vi "thermocouple-calibrate-average.vi"(11 "adam-chassis-all-data-out in":T1) -> (3 "adam-chassis-all-data-out out":T1)   [LabVIEW 2024]
uses:
  adam5000_LLB/controls/adam-5000-all-chassis-data.ctl
  adam5000_LLB/controls/adam-5000-all-module-datas.ctl
  adam5000_LLB/controls/digital-output-cluster.ctl
  adam5000_LLB/controls/digitial-input-cluster.ctl
  adam5000_LLB/controls/analog-output-cluster.ctl
  adam5000_LLB/controls/analog-input-cluster.ctl
  adam5000_LLB/controls/thermocouple-input-cluster.ctl
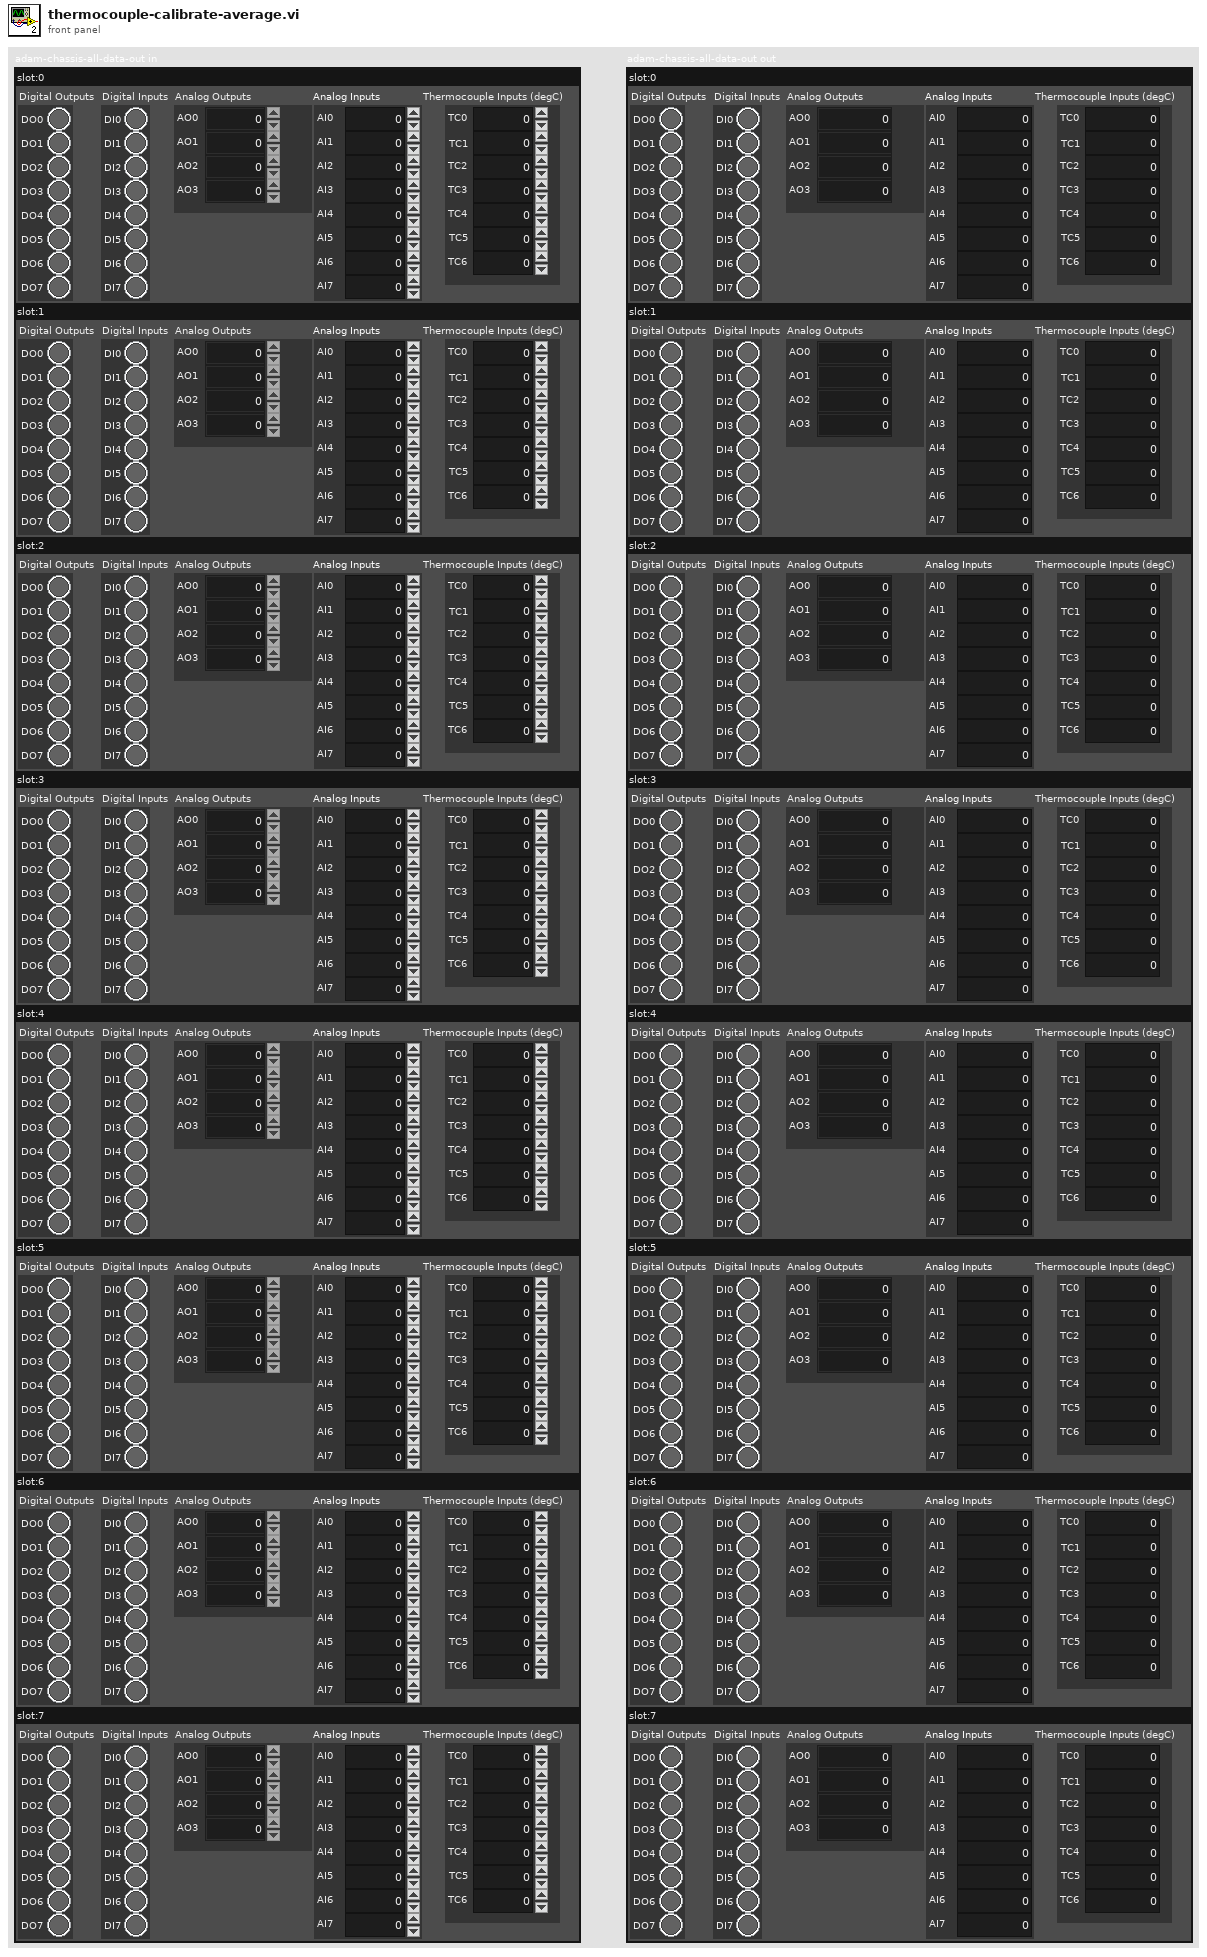
[diagram p1: front panel]
types:
  T1 = typedef "adam-5000-all-chassis-data.ctl" = cluster{"slot:0":T2, "slot:1":T2, "slot:2":T2, "slot:3":T2, "slot:4":T2, "slot:5":T2, "slot:6":T2, "slot:7":T2}
  T2 = typedef "adam-5000-all-module-datas.ctl" = cluster{"Digital Outputs":T3, "Digital Inputs":T4, "Analog Outputs":T5, "Analog Inputs":T6, "Thermocouple Inputs (degC)":T7}
  T3 = typedef "digital-output-cluster.ctl" = cluster{"DO0":bool, "DO1":bool, "DO2":bool, "DO3":bool, "DO4":bool, "DO5":bool, "DO6":bool, "DO7":bool}
  T4 = typedef "digitial-input-cluster.ctl" = cluster{"DI0":bool, "DI1":bool, "DI2":bool, "DI3":bool, "DI4":bool, "DI5":bool, "DI6":bool, "DI7":bool}
  T5 = typedef "analog-output-cluster.ctl" = cluster{"AO0":dbl, "AO1":dbl, "AO2":dbl, "AO3":dbl}
  T6 = typedef "analog-input-cluster.ctl" = cluster{"AI0":dbl, "AI1":dbl, "AI2":dbl, "AI3":dbl, "AI4":dbl, "AI5":dbl, "AI6":dbl, "AI7":dbl}
  T7 = typedef "thermocouple-input-cluster.ctl" = cluster{"TC0":dbl, "TC1":dbl, "TC2":dbl, "TC3":dbl, "TC4":dbl, "TC5":dbl, "TC6":dbl}
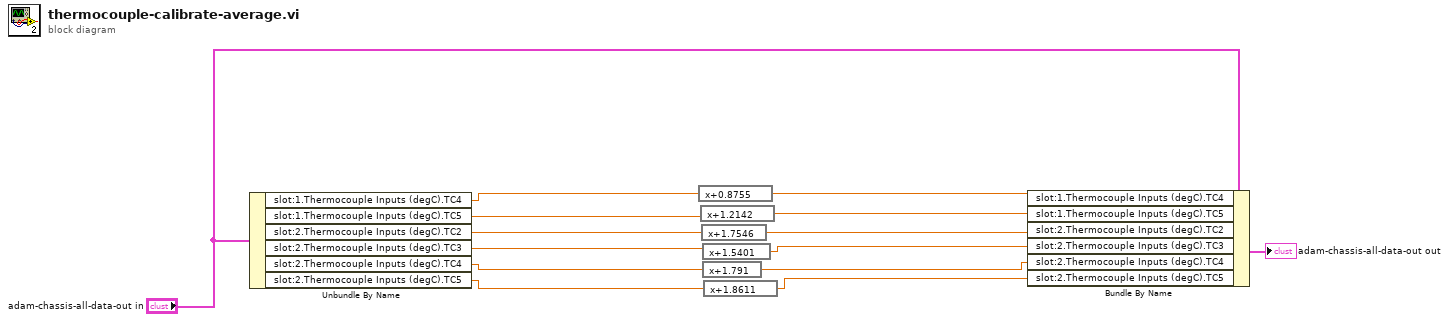
[diagram p0: block diagram]
diagram:
  n1 = Unbundle By Name("adam-chassis-all-data-out in") -> ("slot:1.Thermocouple Inputs (degC).TC4"=w12:dbl, "slot:1.Thermocouple Inputs (degC).TC5"=w10:dbl, "slot:2.Thermocouple Inputs (degC).TC2"=w8:dbl, "slot:2.Thermocouple Inputs (degC).TC3"=w6:dbl, "slot:2.Thermocouple Inputs (degC).TC4"=w4:dbl, "slot:2.Thermocouple Inputs (degC).TC5"=w2:dbl)
  n2 = expression code="x+0.8755"(w12) -> (w11:dbl)
  n3 = expression code="x+1.2142"(w10) -> (w9:dbl)
  n4 = expression code="x+1.7546"(w8) -> (w7:dbl)
  n5 = expression code="x+1.5401"(w6) -> (w5:dbl)
  n6 = expression code="x+1.791"(w4) -> (w3:dbl)
  n7 = expression code="x+1.8611"(w2) -> (w1:dbl)
  n8 = Bundle By Name(cluster="adam-chassis-all-data-out in", "slot:1.Thermocouple Inputs (degC).TC4"=w11, "slot:1.Thermocouple Inputs (degC).TC5"=w9, "slot:2.Thermocouple Inputs (degC).TC2"=w7, "slot:2.Thermocouple Inputs (degC).TC3"=w5, "slot:2.Thermocouple Inputs (degC).TC4"=w3, "slot:2.Thermocouple Inputs (degC).TC5"=w1) -> (→"adam-chassis-all-data-out out":T1)
